vi "write TBM configuration.vi"(8 "error in":errorcluster, 10 "TBM configuration in":refnum<class "TBM configuration.lvclass">, 11 "Tag Bus Web Interface editor node in":refnum<class "Tag Bus Web Interface editor node.lvclass">) -> (0 "error out":errorcluster, 3 "Tag Bus Web Interface editor node out":refnum<class "Tag Bus Web Interface editor node.lvclass">)   [LabVIEW 2013, in "Tag Bus Web Interface editor node.lvclass"]
uses:
  Tag Bus Web Interface editor node.lvclass
  <vilib>/NI/Tag Bus Module Framework/root configuration/TBM configuration.lvclass
  <vilib>/NI/TBM Modules/TBWI/configuration/Tag Bus Web Interface configuration.lvclass
  Tag Bus Web Interface editor node.lvclass/Tag Bus Web Interface editor node.ctl
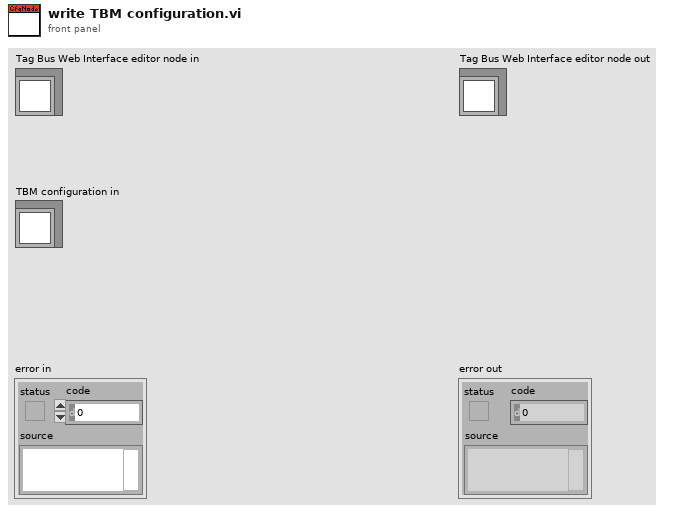
[diagram p1: front panel]
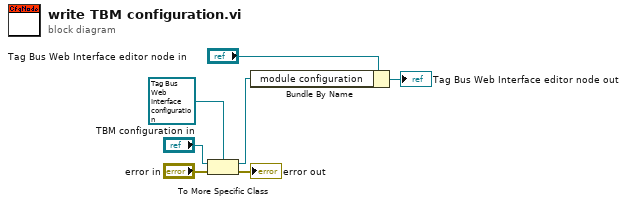
[diagram p0: block diagram]
diagram:
  n1 = To More Specific Class(target class=refnum<class "Tag Bus Web Interface configuration.lvclass"> refnum ("module configuration"), reference="TBM configuration in", error in="error in") -> (specific class reference=w1:refnum<class "Tag Bus Web Interface configuration.lvclass">, error out=→"error out":errorcluster)
  n2 = Bundle By Name(cluster="Tag Bus Web Interface editor node in", "module configuration"=w1) -> (→"Tag Bus Web Interface editor node out":refnum<class "Tag Bus Web Interface editor node.lvclass">)
